vi "Server Start.vi"(8 "error in":errorcluster, 11 "VisionServerRef in":T1) -> (0 "error out":errorcluster, 3 "VisionServerRef out":T1)   [LabVIEW 2016, in "Vision Server.lvclass"]
uses:
  Vision Server.lvclass
  typedef/Vision Server Ref.ctl
  Vision Server.vi
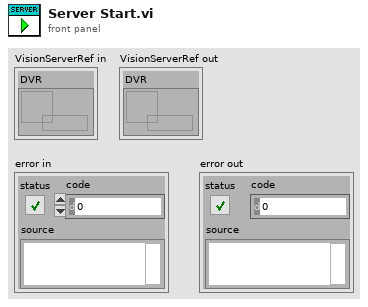
[diagram p1: front panel]
types:
  T1 = typedef "Vision Server.lvclass/Vision Server Ref.ctl" = cluster{"DVR":refnum<data-value>}
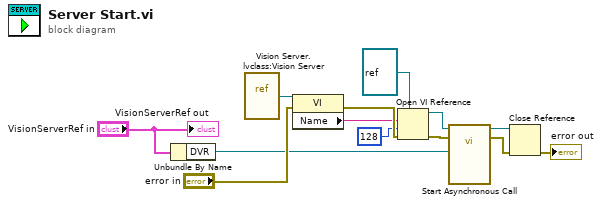
[diagram p0: block diagram]
diagram:
  n1 = Unbundle By Name("VisionServerRef in") -> ("DVR"=w1:refnum<data-value>)
  n2 = vi-ref "Vision Server.lvclass:Vision Server.vi"() -> (w6:refnum<vi>)
  n3 = property class="VI"(reference=w6, error in="error in") -> (error out=w9:errorcluster, "Name"=w3:string)  [unwired: 1 out]
  n4 = Open VI Reference(type specifier VI Refnum (for type only)=refnum<vi> refnum, vi path=w3, options=128, error in (no error)=w9) -> (vi reference=w5:refnum<vi>, error out=w8:errorcluster)  [unwired: 2 in]
  n5 = call-by-ref "Start Asynchronous Call"(reference=w5, error in=w8, "Vision Server"=w1) -> (reference out=w13:refnum<vi>, error out=w11:errorcluster)  [unwired: 10 in, 1 out]
  n6 = Close Reference(reference=w13, error in (no error)=w11) -> (error out=→"error out":errorcluster)
  "VisionServerRef out" <- "VisionServerRef in"
